vi "Add Object.vi"(8 "error in (no error)":errorcluster, 10 "OBJ File":path, 11 "Scene in":refnum<class "Scene.lvclass">) -> (0 "error out":errorcluster, 3 "Scene out":refnum<class "Scene.lvclass">)   [LabVIEW 2020, in "Application.lvlib" / "Scene.lvclass"]
uses:
  Scene.lvclass
  Scene.lvclass/Scene.ctl
  FPGA/Libraries/3D/3D (FPGA).lvlib
  FPGA/Libraries/3D/Vector 3D.ctl
  FPGA/Libraries/3D/Transform.ctl
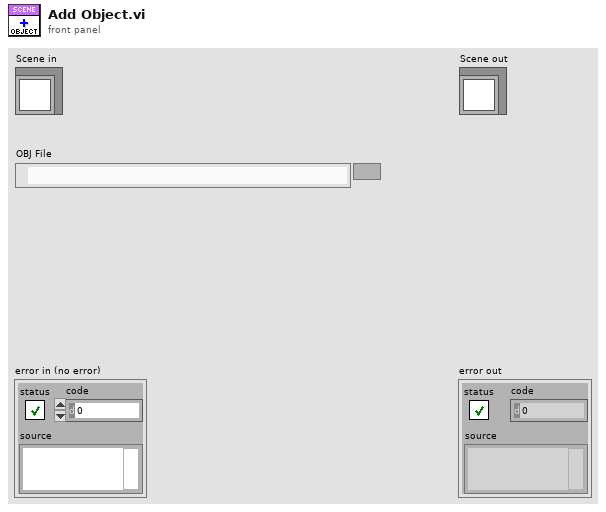
[diagram p1: front panel]
types:
  T1 = typedef "3D (FPGA).lvlib/Transform.ctl" = cluster{"Position":T2, "Rotation":T2, "Scale":T2}
  T2 = typedef "3D (FPGA).lvlib/Vector 3D.ctl" = cluster{"x":sgl, "y":sgl, "z":sgl}
  T3 = typedef "3D (FPGA).lvlib/Object.ctl" = cluster{"Triangles":T4[], "Transform":T1, "Name":string, "Alpha Blending Enabled":bool, "Alpha":dbl, "Turntable Enabled":bool, "Material":T7}
  T4 = typedef "3D (FPGA).lvlib/Triangle.ctl" = cluster{"Vertex 1":T5, "Vertex 2":T5, "Vertex 3":T5, "Alpha":dbl, "Alpha Blending Enabled":bool, "Colour":u32, "Material":T7}
  T5 = typedef "3D (FPGA).lvlib/Vertex.ctl" = cluster{"Position":T2, "UV":T6, "Colour":u32}
  T6 = typedef "Raster (FPGA).lvlib/UV.ctl" = cluster{"u":sgl, "v":sgl}
  T7 = typedef "3D (FPGA).lvlib/Material.ctl" = cluster{"Diffuse Colour":u32, "Texture":T8}
  T8 = typedef "Raster (FPGA).lvlib/Texture.ctl" = cluster{"Pixels":refnum<data-value>, "Size":T9}
  T9 = typedef "Raster (FPGA).lvlib/Rectangle Dimensions.ctl" = cluster{"Width":u32, "Height":u32}
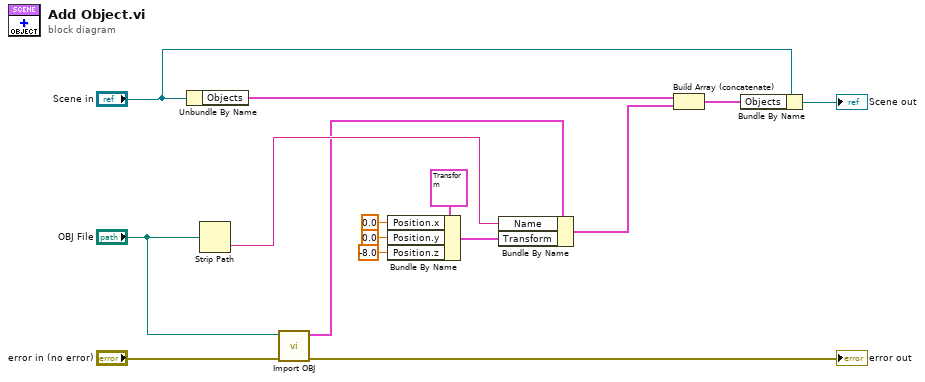
[diagram p0: block diagram]
diagram:
  n1 = Unbundle By Name("Scene in") -> ("Objects"=w8:T3[])
  n2 = Strip Path(path="OBJ File") -> (name=w15:string)  [unwired: 1 out]
  n3 = call "Import OBJ.vi"("error in (no error)"="error in (no error)", "Object"="OBJ File") -> ("error out"=→"error out":errorcluster, "Object"=w1:T3)  [unwired: 8 in]
  n4 = Bundle By Name(cluster=T1 {"Position"={"x"=2.0, "y"=1.0, "z"=-5.0}, "Rotation"={"x"=0.0, "y"=0.0, "z"=0.0}, "Scale"={"x"=0.0, "y"=0.0, "z"=0.0}} ("Transform"), "Position.x"=sgl 0.0, "Position.y"=sgl 0.0, "Position.z"=sgl -8.0) -> (w11:T1)
  n5 = Bundle By Name(cluster=w1, "Name"=w15, "Transform"=w11) -> (w3:T3)
  n6 = Build Array (concatenate)(w8, w3) -> (w4:T3[])
  n7 = Bundle By Name(cluster="Scene in", "Objects"=w4) -> (→"Scene out":refnum<class "Scene.lvclass">)
